vi "GenerateData.vi"(8 "error in (no error)":errorcluster, 11 "DAQ_QPT_Throlab in":refnum<class "DAQ_QPD_Throlab.lvclass">) -> (0 "error out":errorcluster, 2 "DataExchange":T2, 3 "DAQ_QPT_Throlab out":refnum<class "DAQ_QPD_Throlab.lvclass">)   [LabVIEW 2020, in "DAQ_QPD_Throlab.lvlib" / "DAQ_QPD_Throlab.lvclass"]
uses:
  DAQ_QPD_Throlab.lvclass
  Hardware Abstraction Layer/Component/Device/Device/DataExchange.ctl
  Hardware Abstraction Layer/Component/DAQ/DAQ/DAQ.lvclass
  Interface/DataListener/DataListener.lvclass
panel:
  in  "Cluster":T1 {"QPD  Sum" format="%#_13g"; "QPD Voltage Y" format="%#_13g"; "QPD Voltage X" format="%#_13g"}
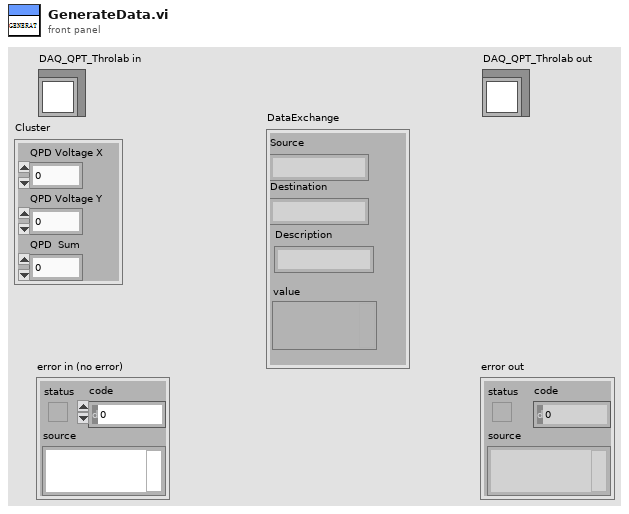
[diagram p1: front panel]
types:
  T1 = cluster{"QPD Voltage X":dbl, "QPD Voltage Y":dbl, "QPD  Sum":dbl}
  T2 = typedef "DataListener.lvclass/DataExchange.ctl" = cluster{"Source":string, "Destination":string, "Description":string, "value":variant}
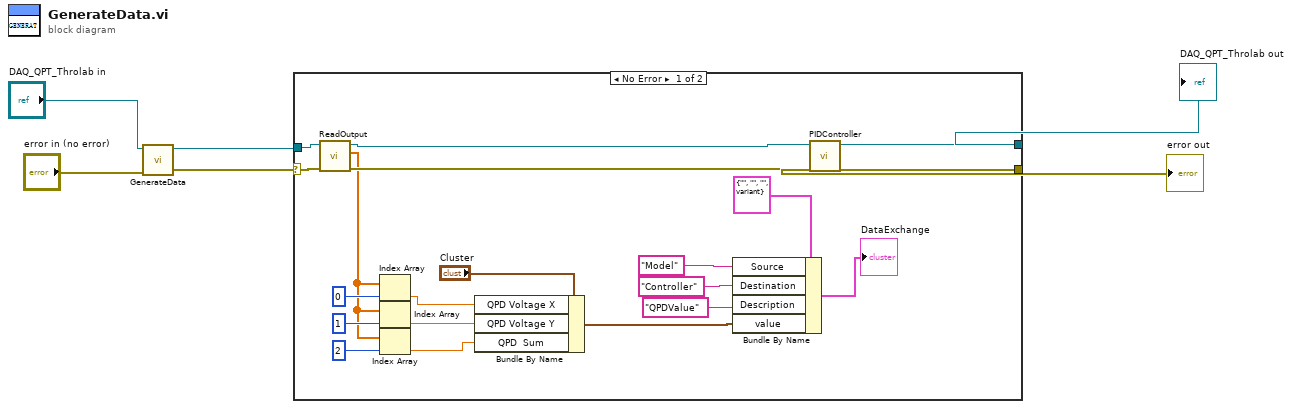
[diagram p0: block diagram]
diagram:
  n1 = call-parent "GenerateData.vi"("error in (no error)"="error in (no error)", "Device in"="DAQ_QPT_Throlab in") -> ("error out"=w3:errorcluster, "Device out"=w4:refnum<class "DAQ_QPD_Throlab.lvclass">)  [unwired: 7 in, 1 out]
  n2 = case shown="No Error" w3 {
    selector: w3 -> [w26 w28]
    tunnel: [w14 w28] -> w1
    tunnel: [w13 w27] -> w2
    tunnel: w4 -> [w24 w27]
    frame No Error {
      n3 = call-dynamic "ReadOutput.vi"("error in (no error)"=w26, "DAQ_QPT_Throlab in"=w24) -> ("error out"=w25:errorcluster, "Output Values"=w19:dbl[], "DAQ_QPT_Throlab out"=w20:refnum<class "DAQ_QPD_Throlab.lvclass">)  [unwired: 7 in]
      n4 = Index Array(array=w19, index=0) -> (element=w18:dbl)
      n5 = Index Array(array=w19, index=1) -> (element=w16:dbl)
      n6 = Index Array(array=w19, index=2) -> (element=w15:dbl)
      n7 = Bundle By Name(cluster="Cluster", "QPD Voltage X"=w18, "QPD Voltage Y"=w16, "QPD  Sum"=w15) -> (w8:T1)
      n8 = Bundle By Name(cluster=T2 {"Source"="", "Destination"="", "Description"="", "value"=variant} ("DataExchange"), "Source"="Model", "Destination"="Controller" ("Type"), "Description"="QPDValue" ("Target"), "value"=w8) -> (→"DataExchange":T2)
      n9 = call-dynamic "PIDController.vi"("error in (no error)"=w25, "DAQ_QPT_Throlab in"=w20) -> ("error out"=w14:errorcluster, "DAQ_QPT_Throlab out"=w13:refnum<class "DAQ_QPD_Throlab.lvclass">)  [unwired: 8 in]
    }
    frame Error {
    }
  }
  "error out" <- w1
  "DAQ_QPT_Throlab out" <- w2
